vi "Pulse waveform generator test.vi"() -> ()   [LabVIEW 2014]
uses:
  <vilib>/measure/NI_MABase.lvlib
panel:
  out "real pulse duration":dbl
  out "Combined":waveform(dbl)(graph)
  out "Pulse waveform":waveform(dbl)(graph)
  out "Sine waveform":waveform(dbl)(graph)
  out "SampClk.Rate":dbl
  in  "Number of Samples":i32=1000
  in  "Cluster":T1={"Waveform Type"=0, "Amplitude"=1.0, "Frequency"=17.0, "Offset"=0.0} {"Frequency" format="%0.2p"; "Amplitude" format="%0.2p"; "Waveform Type" items=["Sine Wave", "Triangle Wave", "Square Wave", "Sawtooth Wave"]}
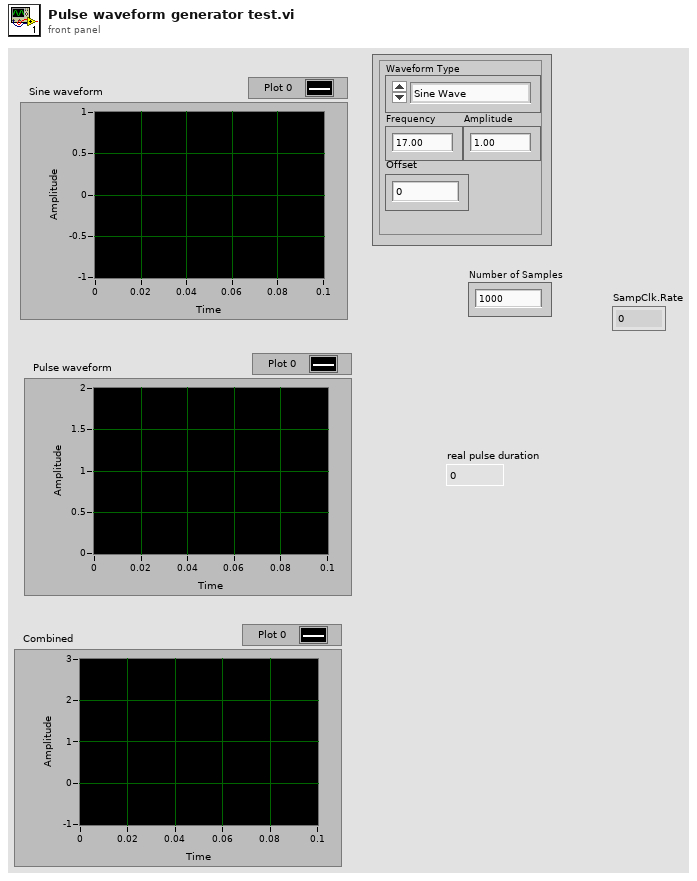
[diagram p1: front panel]
types:
  T1 = cluster{"Waveform Type":u16, "Amplitude":dbl, "Frequency":dbl, "Offset":dbl}
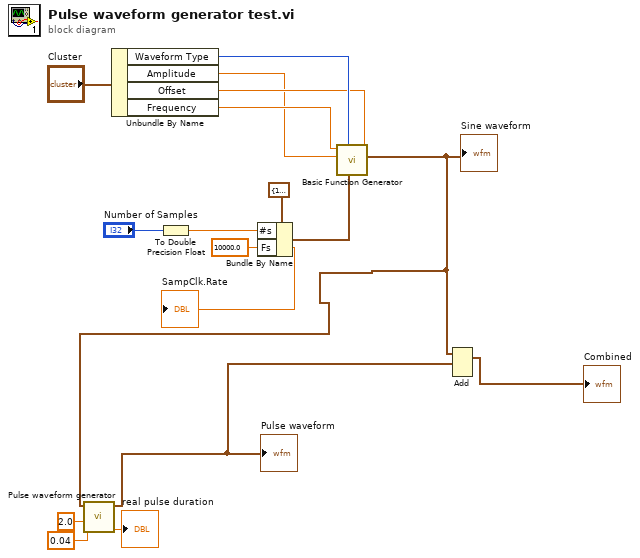
[diagram p0: block diagram]
diagram:
  w9 = 10000.0 ("Fs")
  n1 = Unbundle By Name("Cluster") -> ("Waveform Type"=w15:u16, "Amplitude"=w7:dbl, "Offset"=w14:dbl, "Frequency"=w13:dbl)
  n2 = To Double Precision Float(number="Number of Samples") -> (double precision float=w11:dbl)
  n3 = Bundle By Name(cluster=cluster{"Fs":dbl, "#s":dbl} {"Fs"=1000.0, "#s"=1000.0} ("sampling info"), "#s"=w11, "Fs"=w9) -> (w8:cluster{"Fs":dbl, "#s":dbl})
  n4 = call <vilib>:"Basic Function Generator.vi"("offset"=w14, "sampling info"=w8, "signal type"=w15, "amplitude"=w7, "frequency"=w13) -> ("signal out"=w4:waveform(dbl))  [unwired: 4 in, 2 out]
  "Sine waveform" <- w4
  n5 = call "Pulse waveform generator.vi"("Base waveform"=w4, "Pulse Amplitude"=2.0, "Pulse Duration"=0.04) -> ("Pulse waveform"=w5:waveform(dbl), "real pulse duration"=→"real pulse duration":dbl)  [unwired: 6 in]
  "Pulse waveform" <- w5
  n6 = Add(1:w5, 2:w4) -> (0:→"Combined":waveform(dbl))  [unwired: 1 in, 1 out]
  "SampClk.Rate" <- w9
